vi "Disconnect PV.vi"(8 "error in (no error)":errorcluster, 10 "PV URL":string, 11 "CS++PVMonitor in":refnum<class "CS++PVMonitor.lvclass">) -> (0 "error out":errorcluster, 3 "CS++PVMonitor out":refnum<class "CS++PVMonitor.lvclass">)   [LabVIEW 2012, in "CS++PVMonitor.lvlib" / "CS++PVMonitor.lvclass"]
doc: "Close connection to process variable."
uses:
  CS++PVMonitor.lvclass
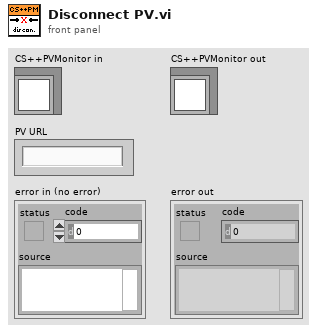
[diagram p1: front panel]
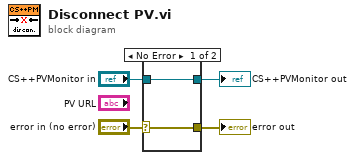
[diagram p0: block diagram]
diagram:
  n1 = case shown="No Error" "error in (no error)" {
    selector: "error in (no error)" -> [w5 w8]
    tunnel: [w5 w8] -> w3
    tunnel: [w6 w7] -> w1
    tunnel: "CS++PVMonitor in" -> [w6 w7]
    frame No Error {
    }
    frame Error {
    }
  }
  "error out" <- w3
  "CS++PVMonitor out" <- w1
